vi "Read String Status.vi"(8 "error in (no error)":errorcluster, 11 "RxTxCamera in":refnum<class "RxTxCamera.lvclass">) -> (0 "error out":errorcluster, 2 "Camera Status":T1, 3 "RxTxCamera out":refnum<class "RxTxCamera.lvclass">)   [LabVIEW 2018, in "RxTxCamera.lvclass"]
doc: "Este VI realiza a leitura da string do status da câmera, retornando um cluster contendo as informações do status da câmera."
uses:
  RxTxCamera.lvclass
  C:/Users/Cliente/Desktop/Software Echarpe/RxTx/RxTx.lvclass
  RxTxCamera.lvclass/RxTxCamera.ctl
  RxTx/RxTx.lvclass/RxTx.ctl
  Construct String Camera Status/Construct String Camera Status.lvclass
  RxTx/RxTx.lvclass
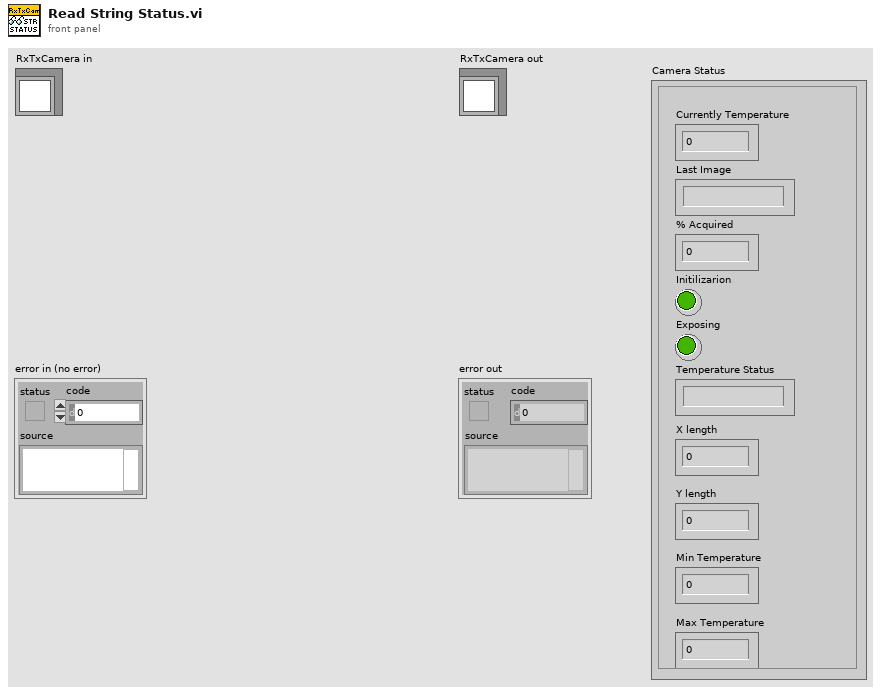
[diagram p1: front panel]
types:
  T1 = cluster{"Currently Temperature":dbl, "Last Image":string, "% Acquired":dbl, "Initilizarion":bool, "Exposing":bool, "Temperature Status":string, "X length":dbl, "Y length":dbl, "Min Temperature":dbl, "Max Temperature":dbl}
  T2 = cluster{"Currently Temperature":dbl, "Last Image":string, "% Acquired":dbl, "Initilization":bool, "Exposing":bool, "Temperature Status":string, "X length":dbl, "Y length":dbl, "Min Temperature":dbl, "Max Temperature":dbl}
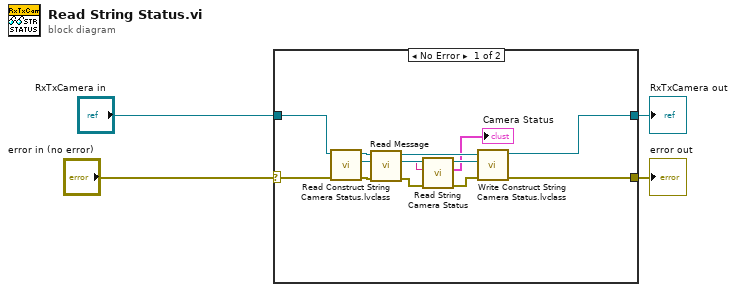
[diagram p0: block diagram]
diagram:
  n1 = case shown="No Error" "error in (no error)" {
    selector: "error in (no error)" -> [w17 w18]
    tunnel: [w15 w18] -> w3
    tunnel: [w14 w19] -> w1
    tunnel: "RxTxCamera in" -> [w13 w19]
    frame No Error {
      n2 = call "Read Construct String Camera Status.lvclass.vi"("error in (no error)"=w17, "RxTxCamera in"=w13) -> ("error out"=w10:errorcluster, "Construct String Camera Status.lvclass"=w12:refnum<class "Construct String Camera Status.lvclass">, "RxTxCamera out"=w9:refnum<class "RxTxCamera.lvclass">)  [unwired: 7 in]
      n3 = call "Read Message.vi"("error in (no error)"=w10, "RxTx in"=w9) -> ("error out"=w7:errorcluster, "Message"=w6:string, "RxTx out"=w8:refnum<class "RxTxCamera.lvclass">)  [unwired: 7 in]
      n4 = call "Read String Camera Status.vi"("error in (no error)"=w7, "String Camera Status"=w6, "Construct String Camera Status in"=w12) -> ("error out"=w16:errorcluster, "Camera Status"=→"Camera Status":T2, "Construct String Camera Status out"=w11:refnum<class "Construct String Camera Status.lvclass">)  [unwired: 6 in]
      n5 = call "Write Construct String Camera Status.lvclass.vi"("error in (no error)"=w16, "Construct String Camera Status.lvclass"=w11, "RxTxCamera in"=w8) -> ("error out"=w15:errorcluster, "RxTxCamera out"=w14:refnum<class "RxTxCamera.lvclass">)  [unwired: 7 in]
    }
    frame Error {
    }
  }
  "error out" <- w3
  "RxTxCamera out" <- w1
